vi "Read UI Constants.vi"(8 "error in (no error)":errorcluster, 11 "CFG File Refnum":T2) -> (0 "error out":errorcluster, 2 "MHL Configuration":T1, 3 "CFG File Refnum out":T2)   [LabVIEW 2015]
uses:
  <vilib>/Utility/config.llb/Config Data RefNum.ctl
  controls/MHL Configuration.ctl
  support/Boiler System Globals.vi
  <vilib>/Utility/config.llb/Read Key (Double).vi
  <vilib>/Utility/config.llb/NI_LVConfig.lvlib
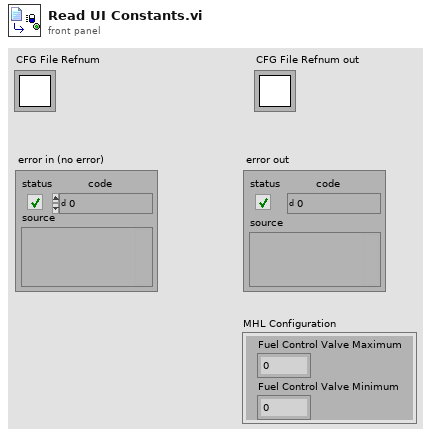
[diagram p1: front panel]
types:
  T1 = typedef "MHL Configuration.ctl" = cluster{"Fuel Control Valve Maximum":dbl, "Fuel Control Valve Minimum":dbl}
  T2 = typedef "NI_LVConfig.lvlib/Config Data RefNum.ctl" = refnum<k1>
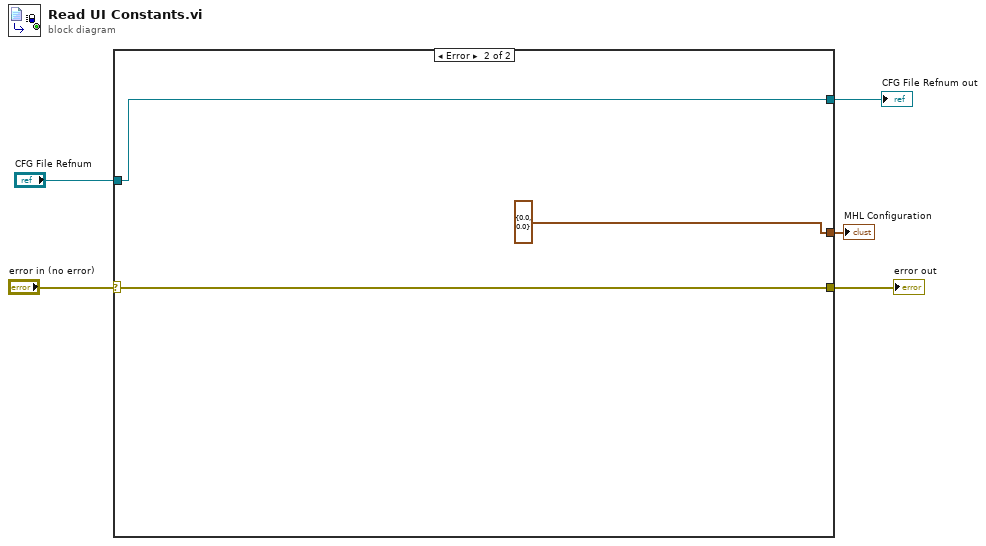
[diagram p0: block diagram]
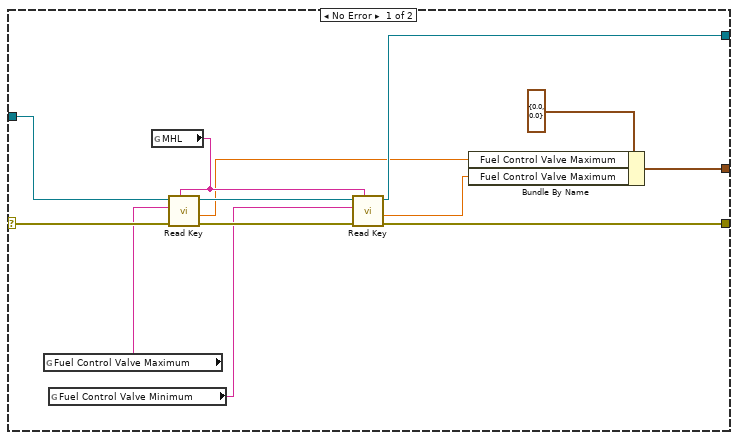
[diagram p2: hidden frame]
diagram:
  n1 = case shown="Error" "error in (no error)" {
    selector: "error in (no error)" -> [w18 w19]
    tunnel: [w17 w19] -> w4
    tunnel: "CFG File Refnum" -> [w13 w21]
    tunnel: [w10 w21] -> w2
    tunnel: [w6 T1 {"Fuel Control Valve Maximum"=0.0, "Fuel Control Valve Minimum"=0.0} ("MHL Configuration")] -> w1
    frame No Error {
      n2 = global read "Boiler System Globals.vi" "Fuel Control Valve Maximum"() -> (w12:string)
      n3 = global read "Boiler System Globals.vi" "Fuel Control Valve Minimum"() -> (w11:string)
      n4 = global read "Boiler System Globals.vi" "MHL"() -> (w14:string)
      n5 = call-poly <vilib>:"Read Key.vi"("section"=w14, "error in (no error)"=w18, "key"=w12, "refnum"=w13) -> ("error out"=w16:errorcluster, "value"=w8:dbl, "refnum out"=w15:T2)  [unwired: 4 in, 1 out]
      n6 = call-poly <vilib>:"Read Key.vi"("section"=w14, "error in (no error)"=w16, "key"=w11, "refnum"=w15) -> ("error out"=w17:errorcluster, "value"=w7:dbl, "refnum out"=w10:T2)  [unwired: 4 in, 1 out]
      n7 = Bundle By Name(cluster=T1 {"Fuel Control Valve Maximum"=0.0, "Fuel Control Valve Minimum"=0.0} ("MHL Configuration"), "Fuel Control Valve Maximum"=w8, "Fuel Control Valve Maximum"=w7) -> (w6:T1)
    }
    frame Error {
    }
  }
  "error out" <- w4
  "CFG File Refnum out" <- w2
  "MHL Configuration" <- w1
